vi "Set Helper.vi"(8 "error in (no error)":errorcluster, 9 "set value":refnum<class "JSON Value.lvclass">, 10 "Array":string[](array[string]), 11 "JSON Value in":refnum<class "JSON Value.lvclass">) -> (0 "error out":errorcluster, 3 "JSON Value out":refnum<class "JSON Value.lvclass">)   [LabVIEW 2016, in "JSON Value.lvclass"]
uses:
  JSON Value.lvclass
  JSON Value.lvclass/JSON Value.ctl
  New JSON Value/New JSON ({}).vi
  Object/Insert Value/Insert Value (Value).vi
  New JSON Value/New JSON (Null).vi
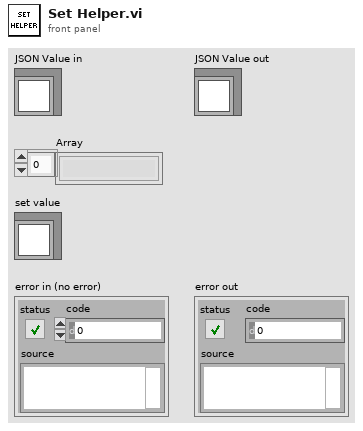
[diagram p1: front panel]
types:
  T1 = typedef "JSON Value.lvclass/JSON Types.ctl" = enum16{"String", "Numeric", "Boolean", "NULL", "Object", "Array"}
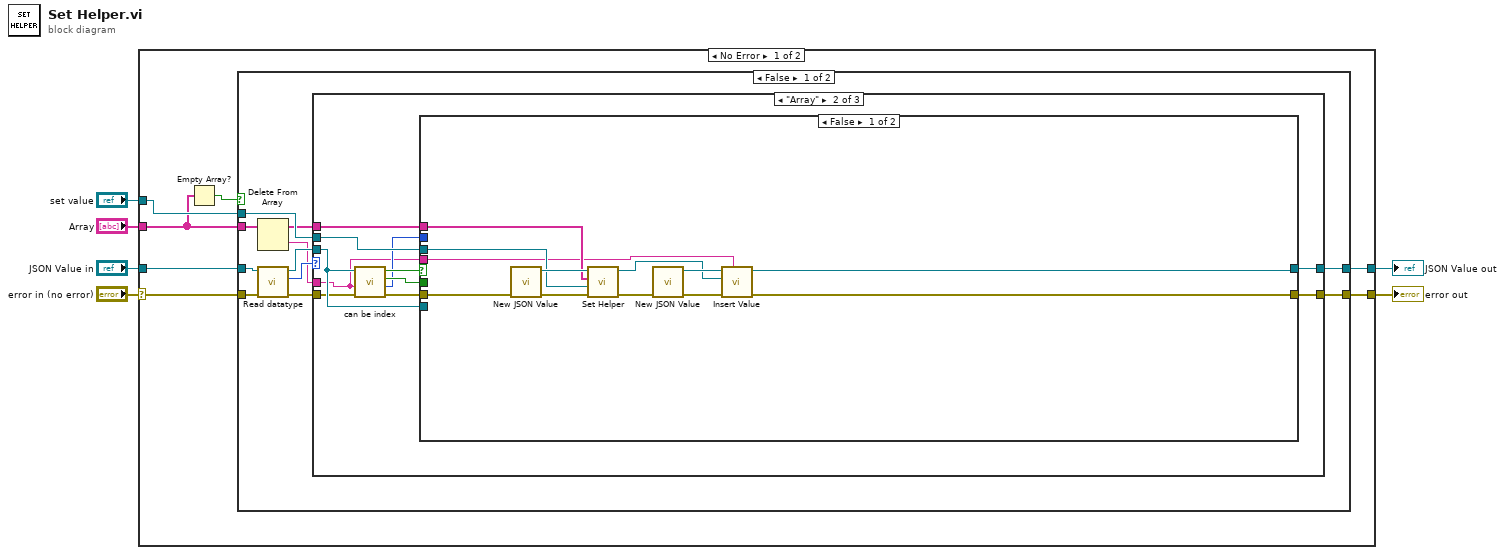
[diagram p0: block diagram]
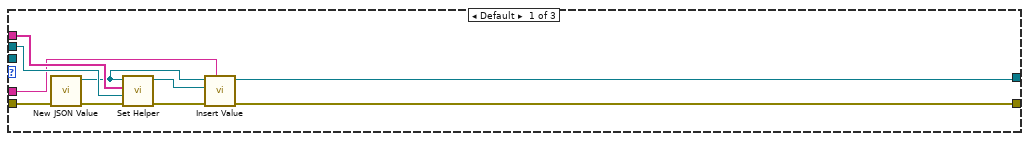
[diagram p2: hidden frame]
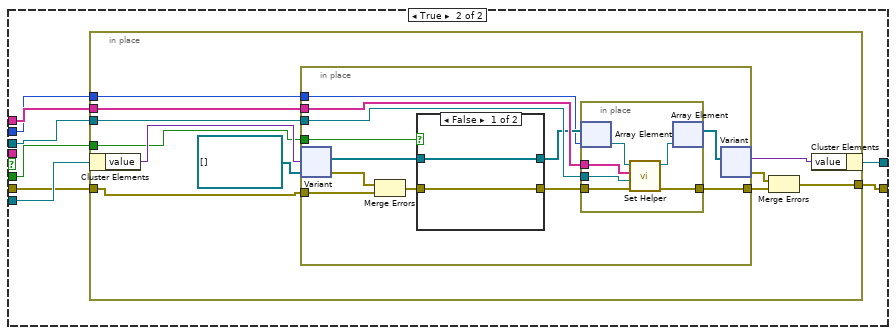
[diagram p3: hidden frame]
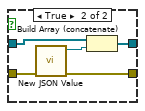
[diagram p4: hidden frame]
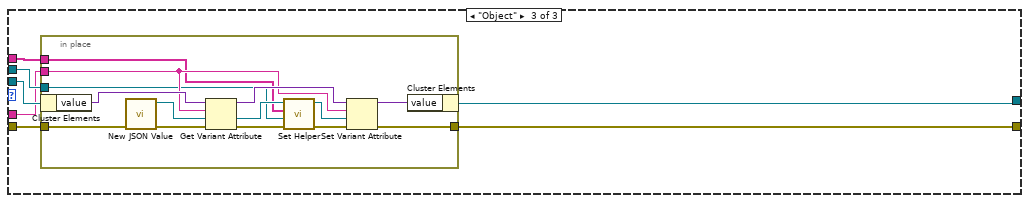
[diagram p5: hidden frame]
diagram:
  n1 = case shown="No Error" "error in (no error)" {
    selector: "error in (no error)" -> [w13 w126]
    tunnel: "JSON Value in" -> [w12 w125]
    tunnel: "Array" -> [w7 _]
    tunnel: [w11 w125] -> w3
    tunnel: "set value" -> [w10 _]
    tunnel: [w9 w126] -> w1
    frame No Error {
      n2 = Empty Array?(array=w7) -> (empty?=w8:bool)
      n3 = case shown="False" w8 {
        tunnel: w13 -> [w24 w123]
        tunnel: w12 -> [w21 _]
        tunnel: w10 -> [w20 w124]
        tunnel: [w18 w124] -> w11
        tunnel: [w17 w123] -> w9
        tunnel: w7 -> [w14 _]
        frame False {
          n4 = Delete From Array(array=w14) -> (deleted portion=w15:string, array with subset deleted=w16:string[])  [unwired: 2 in]
          n5 = call "Read datatype.vi"("error in (no error)"=w24, "JSON Value in"=w21) -> ("error out"=w19:errorcluster, "datatype"=w23:T1, "JSON Value out"=w22:refnum<class "JSON Value.lvclass">)  [unwired: 7 in]
          n6 = case shown="\"Array\"" w23 {
            tunnel: w22 -> [_ w44 w108]
            tunnel: w20 -> [w33 w43 w107]
            tunnel: w19 -> [w32 w41 w106]
            tunnel: [w27 w40 w105] -> w18
            tunnel: [w25 w37 w104] -> w17
            tunnel: w16 -> [w34 w36 w102]
            tunnel: w15 -> [w29 w35 w103]
            frame Default {
              n7 = call-poly "New JSON Value.vi"("error in (no error)"=w32) -> ("error out"=w31:errorcluster, "JSON Value out"=w28:refnum<class "JSON Value.lvclass">)  [unwired: 9 in]
              n8 = call "Set Helper.vi"("error in (no error)"=w31, "set value"=w33, "Array"=w34, "JSON Value in"=w28) -> ("error out"=w26:errorcluster, "JSON Value out"=w30:refnum<class "JSON Value.lvclass">)  [unwired: 6 in]
              n9 = call-poly "Insert Value.vi"("key"=w29, "error in (no error)"=w26, 10:"JSON Value in"=w30, 11:"JSON Value in"=w28) -> ("error out"=w25:errorcluster, "JSON Value out"=w27:refnum<class "JSON Value.lvclass">)  [unwired: 5 in, 1 out]
            }
            frame "Array" {
              n10 = call "can be index.vi"("error in (no error)"=w41, "string"=w35, "JSON Value in"=w44) -> ("error out"=w42:errorcluster, "index"=w38:i32, "last value?"=w39:bool, "valid index?"=w45:bool)  [unwired: 5 in]
              n11 = case shown="False" w45 {
                tunnel: w44 -> [_ w65]
                tunnel: w36 -> [w55 w64]
                tunnel: w43 -> [w54 w63]
                tunnel: w42 -> [w57 w62]
                tunnel: [w49 w61] -> w40
                tunnel: w39 -> [_ w60]
                tunnel: w38 -> [_ w59]
                tunnel: [w48 w58] -> w37
                tunnel: w35 -> [w46 _]
                frame False {
                  n12 = call-poly "New JSON Value.vi"("error in (no error)"=w57) -> ("error out"=w53:errorcluster, "JSON Value out"=w56:refnum<class "JSON Value.lvclass">)  [unwired: 9 in]
                  n13 = call "Set Helper.vi"("error in (no error)"=w53, "set value"=w54, "Array"=w55, "JSON Value in"=w56) -> ("error out"=w47:errorcluster, "JSON Value out"=w51:refnum<class "JSON Value.lvclass">)  [unwired: 6 in]
                  n14 = call-poly "New JSON Value.vi"("error in (no error)"=w47) -> ("error out"=w50:errorcluster, "JSON Value out"=w52:refnum<class "JSON Value.lvclass">)  [unwired: 9 in]
                  n15 = call-poly "Insert Value.vi"("key"=w46, "error in (no error)"=w50, 10:"JSON Value in"=w51, 11:"JSON Value in"=w52) -> ("error out"=w48:errorcluster, "JSON Value out"=w49:refnum<class "JSON Value.lvclass">)  [unwired: 5 in, 1 out]
                }
                frame True {
                  n16 = in-place {
                    in-place-border: w64 -> [w74]
                    in-place-border: w63 -> [w73]
                    in-place-border: w62 -> [w72]
                    in-place-border: w60 -> [w70]
                    in-place-border: w59 -> [w69]
                    in-place-border: [w66] -> w58
                    n17 = in-place-cluster #1(w65) -> ("value"=w76:variant)
                    n18 = in-place {
                      in-place-border: w74 -> [w88]
                      in-place-border: w73 -> [w87]
                      in-place-border: w72 -> [w80]
                      in-place-border: w70 -> [w85]
                      in-place-border: w69 -> [w82]
                      in-place-border: [w77] -> w68
                      n19 = in-place-variant #2(w76, refnum<class "JSON Value.lvclass">[] [] ("JSON Value out")) -> (w84:refnum<class "JSON Value.lvclass">[], w81:errorcluster)
                      n20 = Merge Errors(w81, w80) -> (w79:errorcluster)
                      n21 = case shown="False" w85 {
                        tunnel: w84 -> [w90 w95]
                        tunnel: [w90 w93] -> w83
                        tunnel: w79 -> [w89 w92]
                        tunnel: [w89 w91] -> w78
                        frame False {
                        }
                        frame True {
                          n22 = call-poly "New JSON Value.vi"("error in (no error)"=w92) -> ("error out"=w91:errorcluster, "JSON Value out"=w94:refnum<class "JSON Value.lvclass">)  [unwired: 9 in]
                          n23 = Build Array (concatenate)(w95, w94) -> (w93:refnum<class "JSON Value.lvclass">[])
                        }
                      }
                      n24 = in-place {
                        in-place-border: w88 -> [w99]
                        in-place-border: w87 -> [w98]
                        in-place-border: w78 -> [w97]
                        in-place-border: [w96] -> w77
                        n25 = in-place-array #3(w83, w82) -> (w101:refnum<class "JSON Value.lvclass">)
                        n26 = call "Set Helper.vi"("error in (no error)"=w97, "set value"=w98, "Array"=w99, "JSON Value in"=w101) -> ("error out"=w96:errorcluster, "JSON Value out"=w100:refnum<class "JSON Value.lvclass">)  [unwired: 6 in]
                        n27 = in-place-array #3(w100) -> (w86:refnum<class "JSON Value.lvclass">[])  [unwired: 1 out]
                      }
                      n28 = in-place-variant #2(w86) -> (w71:variant, w67:errorcluster)
                    }
                    n29 = Merge Errors(w67, w68) -> (w66:errorcluster)
                    n30 = in-place-cluster #1("value"=w71) -> (w61:refnum<class "JSON Value.lvclass">)
                  }
                }
              }
            }
            frame "Object" {
              n31 = in-place {
                in-place-border: w102 -> [w116]
                in-place-border: w107 -> [w115]
                in-place-border: w106 -> [w114]
                in-place-border: [w110] -> w104
                in-place-border: w103 -> [w117]
                n32 = in-place-cluster #4(w108) -> ("value"=w122:variant)
                n33 = call-poly "New JSON Value.vi"("error in (no error)"=w114) -> ("error out"=w113:errorcluster, "JSON Value out"=w121:refnum<class "JSON Value.lvclass">)  [unwired: 9 in]
                n34 = Get Variant Attribute(Variant=w122, name=w117, default value (empty Variant)=w121, error in=w113) -> (duplicate Variant=w120:variant, value=w119:refnum<class "JSON Value.lvclass">, error out=w112:errorcluster)  [unwired: 1 out]
                n35 = call "Set Helper.vi"("error in (no error)"=w112, "set value"=w115, "Array"=w116, "JSON Value in"=w119) -> ("error out"=w111:errorcluster, "JSON Value out"=w118:refnum<class "JSON Value.lvclass">)  [unwired: 6 in]
                n36 = Set Variant Attribute(Variant=w120, name=w117, value=w118, error in=w111) -> (Variant out=w109:variant, error out=w110:errorcluster)  [unwired: 1 out]
                n37 = in-place-cluster #4("value"=w109) -> (w105:refnum<class "JSON Value.lvclass">)
              }
            }
          }
        }
        frame True {
        }
      }
    }
    frame Error {
    }
  }
  "JSON Value out" <- w3
  "error out" <- w1
